vi "Get_States_and_Data.vi"(0 "Coffee_Machine_Data":T2={"Backend_Data"={"Level"={"Water_Level"=0.0, "Bean_Level"=0.0, "Milk_Level"=0.0}, "Total_Cups"=0.0}, "Selector"={"Select_Bevarage"=0, "Cup"=FALSE, "Carafe"=FALSE}, "Cup_Unit"=5.0, "Carafe_Unit"=20.0, "Ingreedient_File_PAth"=path "", "Process_Needed"=[], "Indredient_Needed"=[], "Time_Needed"=[], "State_and_Data"={"State"="", "Data"=variant}, "Chamber_Quantity"=0.0, "Dispenser_Quantiry"=0.0, "Dispaly"={"Low_Water"=FALSE, "Low_Bean"=FALSE, "Low_Milk"=FALSE, "Chamber"=0.0, "Dispenser"=0.0, "Purging"=FALSE, "Heating"=FALSE, "Grinding"=FALSE, "Brewing"=FALSE, "Dispensing"=FALSE, "Elapsed_Time"=0.0}} {"Dispaly"."Dispenser" scale=0.0..80.0; "Dispaly"."Chamber" scale=0.0..80.0; "Backend_Data"."Level"."Milk_Level" scale=0.0..100.0; "Backend_Data"."Level"."Bean_Level" scale=0.0..100.0; "Backend_Data"."Level"."Water_Level" scale=0.0..100.0; "Selector"."Select_Bevarage" scale=0.0..2.0}) -> (4 "States_and_Data":T1[](array[typedef]))   [LabVIEW 2023]
uses:
  Controls/Coffee_Machine_Data.ctl
  Controls/Quantity_Data.ctl
  Controls/Select_Preference.ctl
  Controls/State_and_Data.ctl
  Controls/Coffee_Machine_Dispaly.ctl
panel:
  # "COFFEE MACHINE"
  # "Backend Control Panel"
  # "Coffee"
  # "Latte"
  # "Hot Water"
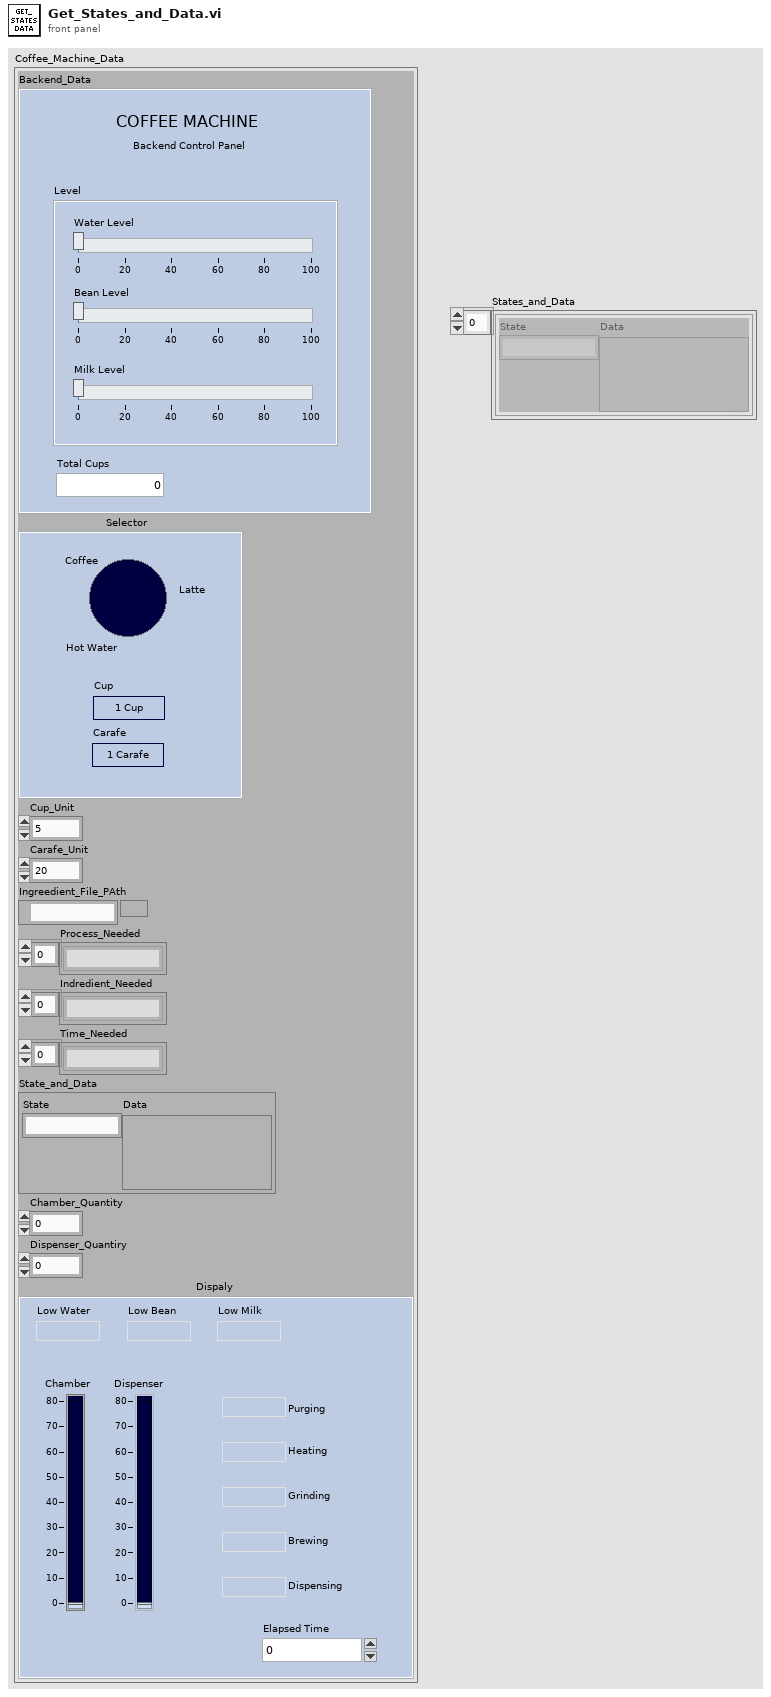
[diagram p1: front panel]
types:
  T1 = typedef "State_and_Data.ctl" = cluster{"State":string, "Data":variant}
  T2 = typedef "Coffee_Machine_Data.ctl" = cluster{"Backend_Data":T3, "Selector":T4, "Cup_Unit":dbl, "Carafe_Unit":dbl, "Ingreedient_File_PAth":path, "Process_Needed":string[], "Indredient_Needed":string[], "Time_Needed":string[], "State_and_Data":T1, "Chamber_Quantity":dbl, "Dispenser_Quantiry":dbl, "Dispaly":T5}
  T3 = typedef "Quantity_Data.ctl" = cluster{"Level":cluster{"Water_Level":dbl, "Bean_Level":dbl, "Milk_Level":dbl}, "Total_Cups":dbl}
  T4 = typedef "Select_Preference.ctl" = cluster{"Select_Bevarage":i32, "Cup":bool, "Carafe":bool}
  T5 = typedef "Coffee_Machine_Dispaly.ctl" = cluster{"Low_Water":bool, "Low_Bean":bool, "Low_Milk":bool, "Chamber":dbl, "Dispenser":dbl, "Purging":bool, "Heating":bool, "Grinding":bool, "Brewing":bool, "Dispensing":bool, "Elapsed_Time":dbl}
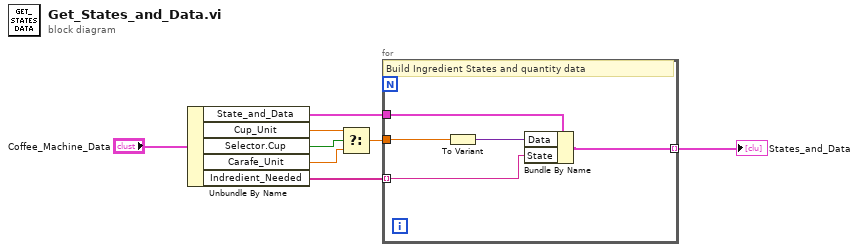
[diagram p0: block diagram]
diagram:
  n1 = Unbundle By Name("Coffee_Machine_Data") -> ("State_and_Data"=w3:T1, "Cup_Unit"=w7:dbl, "Selector.Cup"=w6:bool, "Carafe_Unit"=w8:dbl, "Indredient_Needed"=w1:string[])
  n2 = Select(t=w7, s=w6, f=w8) -> (s? t:f=w5:dbl)
  n3 = for {
    tunnel: w1 -> [w12] mode=indexing
    tunnel: w5 -> [w11]
    tunnel: w3 -> [w13]
    tunnel: [w9] -> w2 mode=indexing
    # "Build Ingredient States and quantity data"
    n4 = To Variant(anything=w11) -> (Variant=w10:variant)
    n5 = Bundle By Name(cluster=w13, "Data"=w10, "State"=w12) -> (w9:T1)
  }
  "States_and_Data" <- w2
